vi "test11-RegisterStatusFromNonCSM_State.vi"(8 "error in (no error)":errorcluster, 11 "TestCase in":refnum<class "testcase-CSMBroadcast.lvclass">) -> (0 "error out":errorcluster, 3 "TestCase out":refnum<class "testcase-CSMBroadcast.lvclass">)   [LabVIEW 2017, in "testcase-CSMBroadcast.lvclass"]
uses:
  testcase-CSMBroadcast.lvclass
  <vilib>/addons/_JKI Toolkits/VI Tester/TestCase.llb/TestCase.lvclass
  src/user.lib/_NEVSTOP/Communicable State Machine(CSM)/Communicable State Machine.lvlib
  CSM/CSM-Testcase.lvlib
  C:/Program Files (x86)/National Instruments/LabVIEW 2017/vi.lib/addons/_JKI Toolkits/VI Tester/TestCase.llb/TestCase.lvclass
panel:
  out "LoopCount":i32
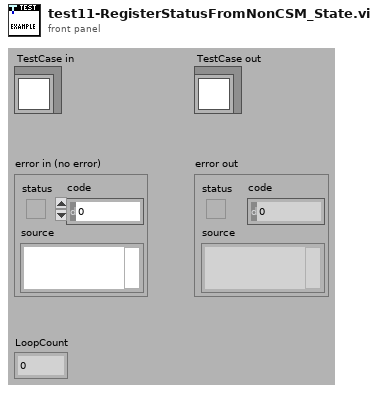
[diagram p1: front panel]
types:
  T1 = cluster{"ModuleName":string, "Status":string, "Arguments":string}
  T2 = cluster{"cluster":cluster{"ModuleName":string, "Status":string, "Arguments":string}}
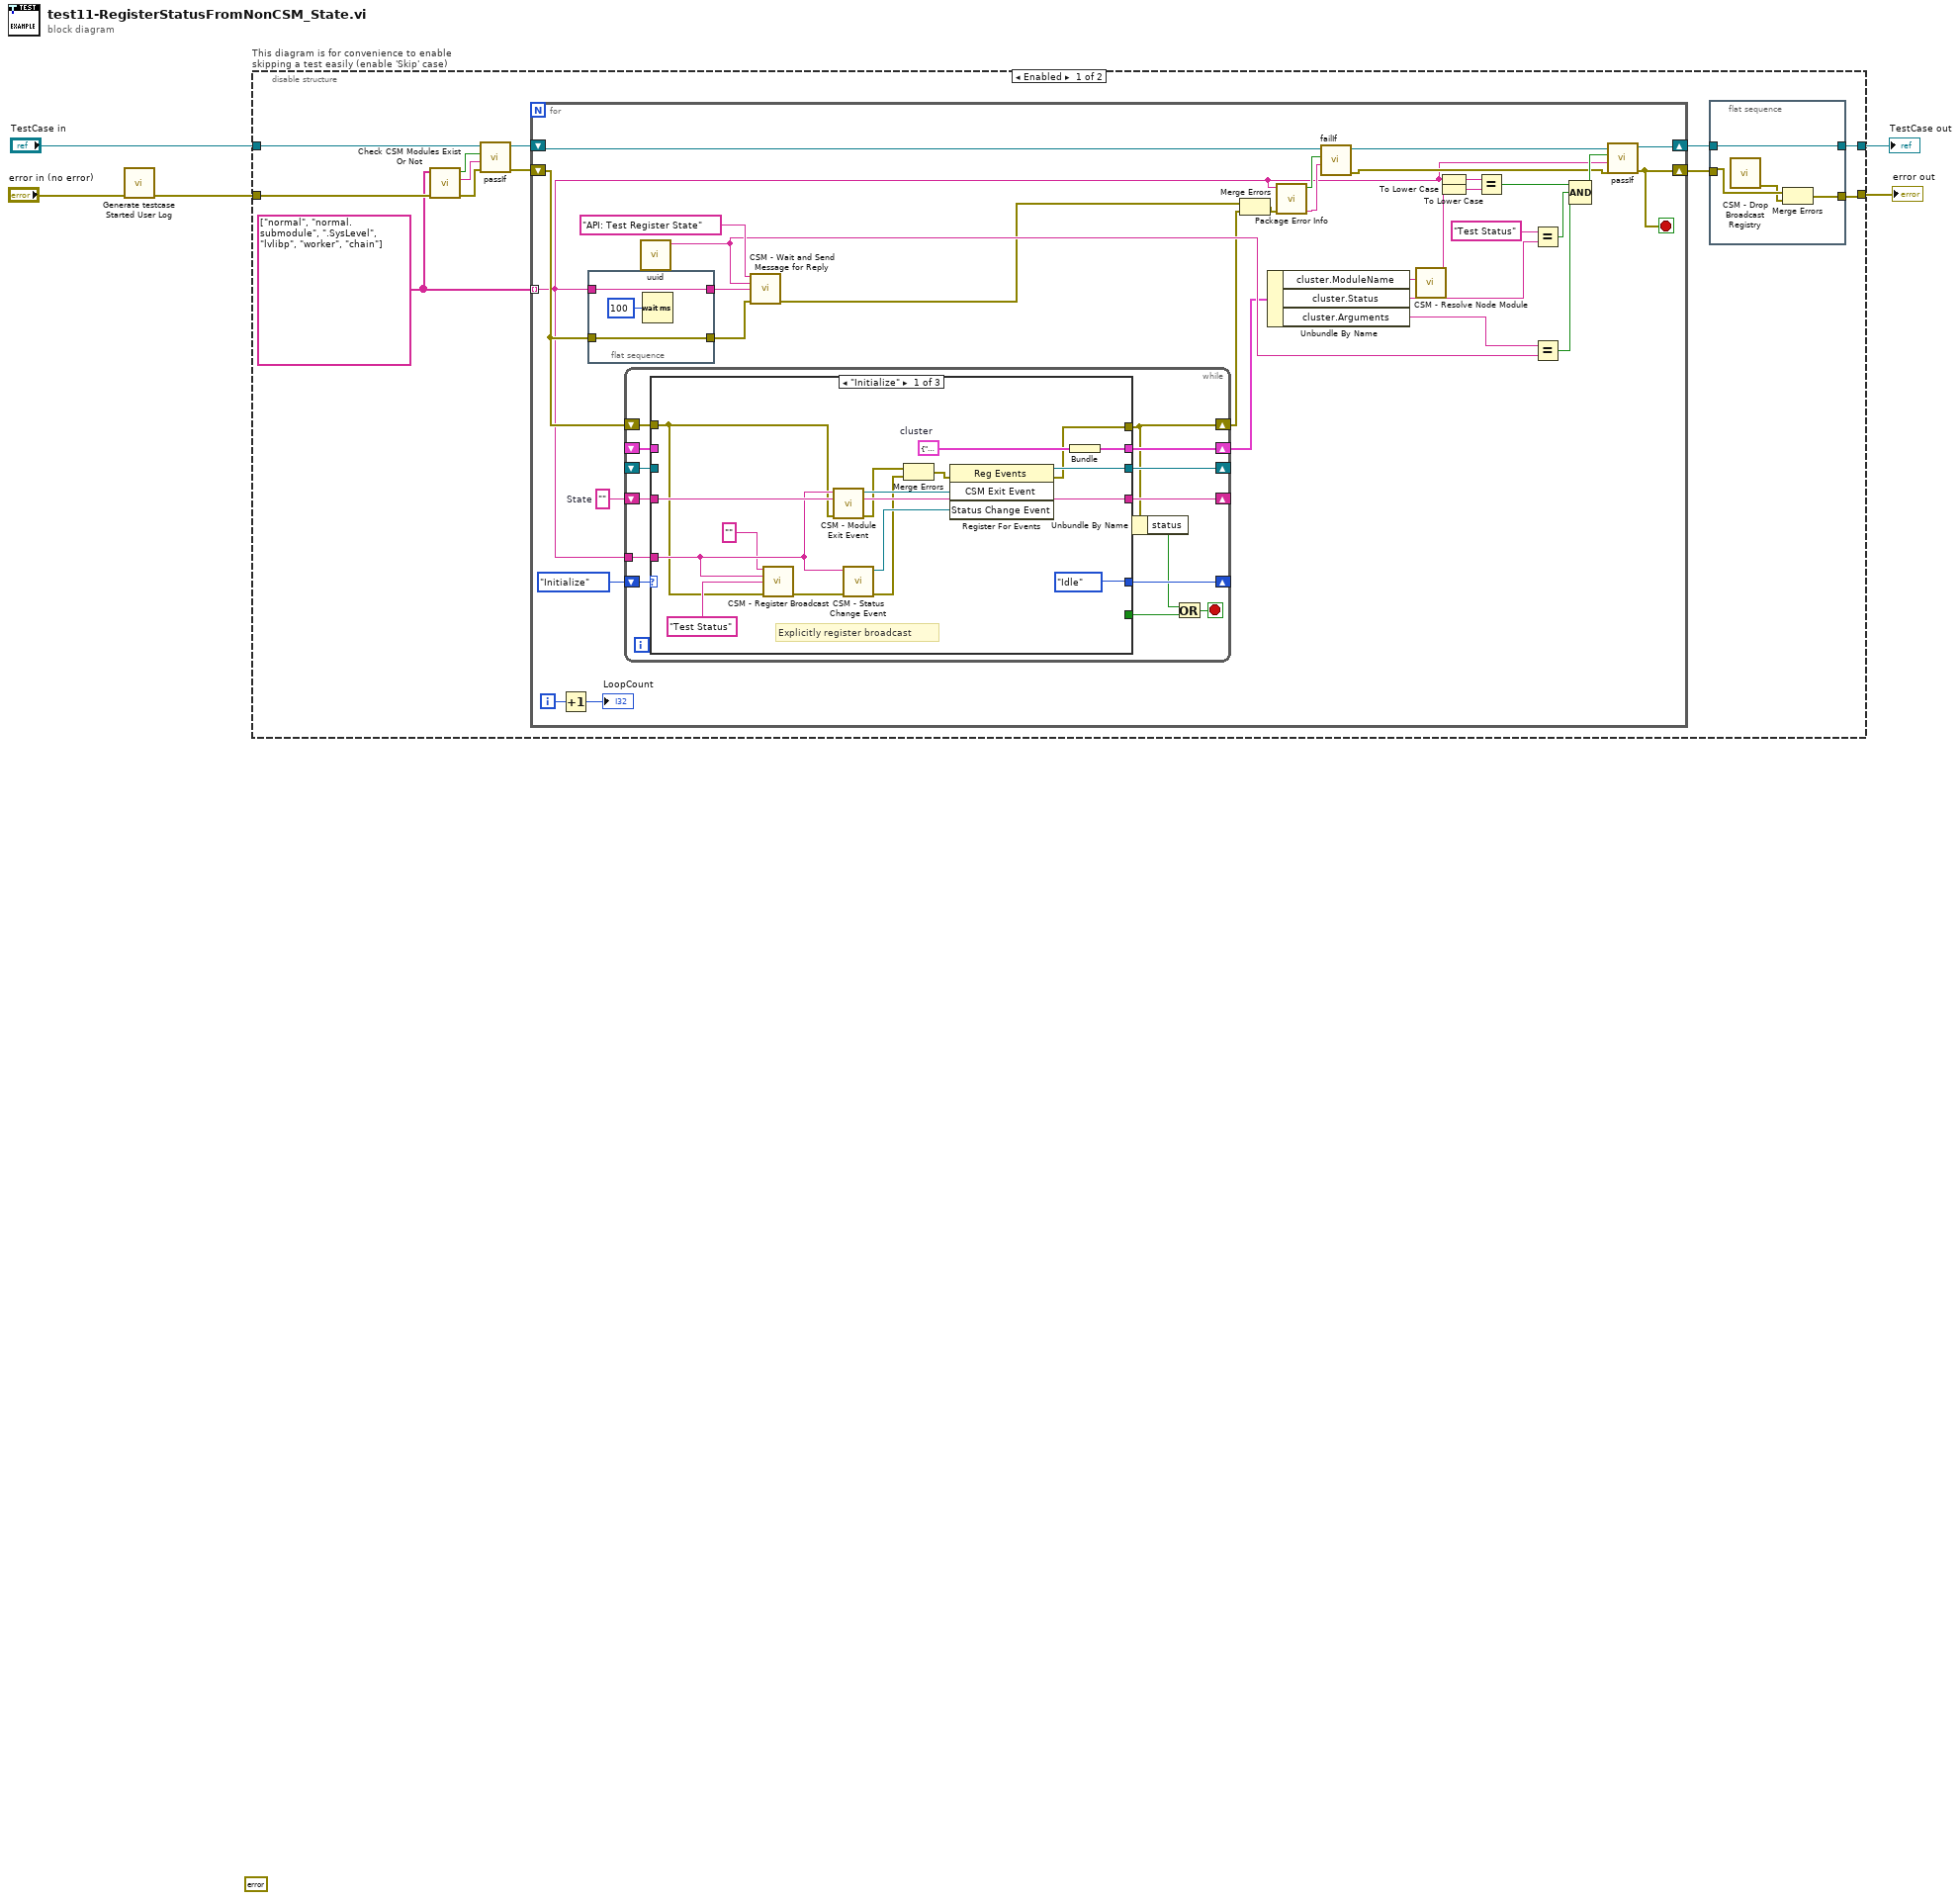
[diagram p0: block diagram]
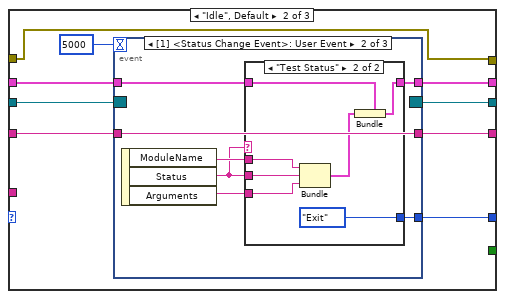
[diagram p2: hidden frame]
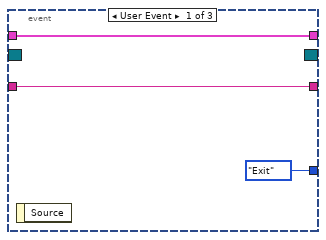
[diagram p3: hidden frame]
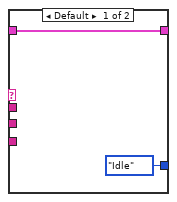
[diagram p4: hidden frame]
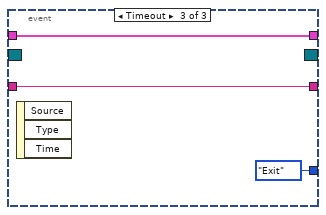
[diagram p5: hidden frame]
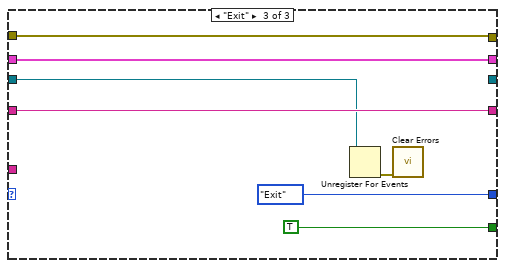
[diagram p6: hidden frame]
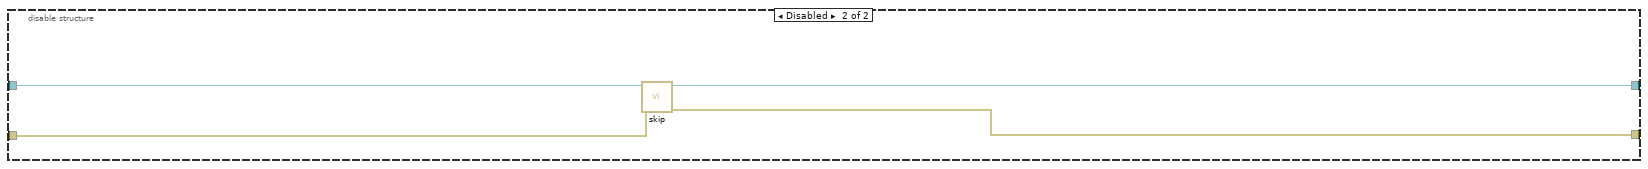
[diagram p7: hidden frame]
diagram:
  (unwired) errorcluster {"status"=FALSE, "code"=0, "source"=""} ("error out")
  n1 = call "Generate testcase Started User Log.vi"("Error In"="error in (no error)") -> ("error out"=w1:errorcluster)  [unwired: 10 in]
  n2 = disable-structure "This diagram is for convenience to enable skipping a test easily (enable 'Skip' case)" shown="Enabled" {
    disable-tunnel: "TestCase in" -> [w13 w128]
    disable-tunnel: [w7 w126] -> w3
    disable-tunnel: [w17 w127] -> w2
    disable-tunnel: w1 -> [w10 w125]
    frame Enabled {
      w9 = string[] ["normal", "normal.submodule", ".SysLevel", "lvlibp", "worker", "chain"]
      n3 = call "Check CSM Modules Exist Or Not.vi"("error in"=w10, "CSM names in"=w9) -> ("error out"=w14:errorcluster, "Debug string"=w15:string, "All Modules Exist?"=w16:bool)  [unwired: 7 in]
      n4 = call-dynamic "passIf.vi"("error in (no error)"=w14, "message (\"\")"=w15, "pass"=w16, "TestCase in"=w13) -> ("error out"=w11:errorcluster, "TestCase out"=w12:refnum<class "testcase-CSMBroadcast.lvclass">)  [unwired: 6 in]
      n5 = for {
        shift-right: [w45] -> w8
        shift-left: w12 -> [w29]
        tunnel: w9 -> [w24] mode=indexing
        shift-right: [w38] -> w6
        shift-left: w11 -> [w31]
        i -> [w40]
        stop <- w38 stop-if-true
        w52 = ""  # State
        n6 = Increment(x=w40) -> (x+1=→"LoopCount":i32)
        n7 = flat-sequence {
          tunnel: w24 -> [w56]
          tunnel: [w56] -> w50
          tunnel: w31 -> [w54]
          tunnel: [w54] -> w32
          frame #0 {
            n8 = Wait (ms)(milliseconds to wait=u32 100) -> ()  [unwired: 1 out]
          }
        }
        n9 = while {
          shift-right: [w69] -> _
          shift-left: enum16{"Idle", "Initialize", "Exit"}."Initialize" -> [w70]
          shift-right: [w67] -> _
          shift-left: w52 -> [w68]
          shift-right: [w66] -> _
          shift-left: _ -> [w65]
          shift-right: [w64] -> w37
          shift-left: _ -> [w63]
          tunnel: w24 -> [w62]
          shift-right: [w58] -> w26
          shift-left: w31 -> [w61]
          stop <- w60 stop-if-true
          n10 = case shown="\"Initialize\"" w70 {
            tunnel: [enum16{"Idle", "Initialize", "Exit"}."Idle" w95 enum16{"Idle", "Initialize", "Exit"}."Exit"] -> w69
            tunnel: [_ _ TRUE] -> w59
            tunnel: w68 -> [w85 w93 w122]
            tunnel: [w85 w94 w122] -> w67
            tunnel: [w83 w91 _] -> w66
            tunnel: w65 -> [_ w92 w121]
            tunnel: [w82 w89 w119] -> w64
            tunnel: w63 -> [_ w90 w119]
            tunnel: w62 -> [w76 _ _]
            tunnel: w61 -> [w73 w87 w118]
            tunnel: [w71 w87 w118] -> w58
            frame "Initialize" {
              w80 = T1 {"ModuleName"="", "Status"="", "Arguments"=""}  # cluster
              # "Explicitly register broadcast"
              n11 = call "CSM - Register Broadcast.vi"("CSM Name(Empty for Broadcast Event)"="", "Source CSM Name (* as Default)"=w76, "Trigger"="Test Status" ("State"), "Error In"=w73) -> ("error out"=w77:errorcluster)  [unwired: 10 in, 1 out]
              n12 = call "CSM - Module Exit Event.vi"("Error In"=w73, "Name (\"\" to Use UUID) In"=w76) -> ("error out"=w79:errorcluster, "CSM Exit Event"=w84:refnum<user-event>)  [unwired: 7 in, 1 out]
              n13 = call "CSM - Status Change Event.vi"("Error In"=w77, "CSM Module"=w76) -> ("error out"=w78:errorcluster, "Status Change Event"=w81:refnum<user-event>)  [unwired: 7 in, 1 out]
              n14 = Merge Errors(w79, w78) -> (w72:errorcluster)
              n15 = register-events(error in=w72, w84, w81) -> (reference out=w83:refnum<event-registration>, error out=w71:errorcluster)  [unwired: 1 in]
              n16 = Bundle("cluster"=w80) -> (w82:T2)  [unwired: 1 in]
            }
            frame "Idle", Default {
              n17 = event shown="[1] <Status Change Event>: User Event" {
                selector: w92 -> [_ _ _]
                dyn-events: [_ _ _] -> w91
                timeout: 5000 -> [_ _ _]
                tunnel: [enum16{"Idle", "Initialize", "Exit"}."Exit" w104 enum16{"Idle", "Initialize", "Exit"}."Exit"] -> w95
                tunnel: w93 -> [w98 w105 w117]
                tunnel: [w98 w105 w117] -> w94
                tunnel: w90 -> [w96 w101 w116]
                tunnel: [w96 w100 w116] -> w89
                event User Event {
                  n18 = event-data() -> ()  [unwired: 1 in, 1 out]
                }
                event User Event {
                  n19 = event-data() -> ("ModuleName"=w103:string, "Status"=w99:string, "Arguments"=w102:string)  [unwired: 1 in]
                  n20 = case shown="\"Test Status\"" w99 {
                    tunnel: [enum16{"Idle", "Initialize", "Exit"}."Idle" enum16{"Idle", "Initialize", "Exit"}."Exit"] -> w104
                    tunnel: w103 -> [_ w113]
                    tunnel: w99 -> [_ w112]
                    tunnel: w102 -> [_ w111]
                    tunnel: w101 -> [w107 w110]
                    tunnel: [w107 w108] -> w100
                    frame Default {
                    }
                    frame "Test Status" {
                      n21 = Bundle("ModuleName"=w113, "Status"=w112, "Arguments"=w111) -> (w109:T1)  [unwired: 1 in]
                      n22 = Bundle(cluster=w110, "cluster"=w109) -> (w108:T2)
                    }
                  }
                }
                event Timeout {
                  n23 = event-data() -> ()  [unwired: 1 in, 3 out]
                }
              }
            }
            frame "Exit" {
              n24 = Unregister For Events(event registration refnum=w121) -> (error out=w120:errorcluster)  [unwired: 1 in]
              n25 = call <vilib>:"Clear Errors.vi"("error in (no error)"=w120) -> ()  [unwired: 5 in, 2 out]
            }
          }
          n26 = Unbundle By Name(w58) -> ("status"=w57:bool)
          n27 = Or(x=w57, y=w59) -> (x .or. y?=w60:bool)
        }
        n28 = call "uuid.vi"() -> ("UUID"=w47:string)  [unwired: 11 in]
        n29 = call "CSM - Wait and Send Message for Reply.vi"("State"="API: Test Register State", "Arguments (\"\")"=w47, "Target Module"=w50, "Error In (No Error)"=w32) -> ("error out"=w22:errorcluster)  [unwired: 8 in, 3 out]
        n30 = Merge Errors(w22, w26) -> (w23:errorcluster)
        n31 = Unbundle By Name(w37) -> ("cluster.ModuleName"=w35:string, "cluster.Status"=w48:string, "cluster.Arguments"=w46:string)
        n32 = call "Package Error Info.vi"("error in"=w23, "String in"=w24) -> ("packed error info out"=w27:string, "error status"=w30:bool)  [unwired: 8 in]
        n33 = call-dynamic "failIf.vi"("message (\"\")"=w27, "fail"=w30, "TestCase in"=w29) -> ("error out"=w25:errorcluster, "TestCase out"=w28:refnum<class "testcase-CSMBroadcast.lvclass">)  [unwired: 7 in]
        n34 = call "CSM - Resolve Node Module.vi"("Node Name"=w35) -> ("CSM Module Name"=w33:string)  [unwired: 10 in]
        n35 = To Lower Case(string=w24) -> (all lower case string=w36:string)
        n36 = To Lower Case(string=w33) -> (all lower case string=w34:string)
        n37 = Equal?(x=w36, y=w34) -> (x = y?=w44:bool)
        n38 = Equal?(x="Test Status" ("State"), y=w48) -> (x = y?=w43:bool)
        n39 = Equal?(x=w46, y=w47) -> (x = y?=w42:bool)
        n40 = Compound Arithmetic op=AND(w44, w43, w42) -> (w41:bool)
        n41 = call-dynamic "passIf.vi"("error in (no error)"=w25, "message (\"\")"=w24, "pass"=w41, "TestCase in"=w28) -> ("error out"=w38:errorcluster, "TestCase out"=w45:refnum<class "testcase-CSMBroadcast.lvclass">)  [unwired: 6 in]
      }
      n42 = flat-sequence {
        tunnel: w6 -> [w21]
        tunnel: [w20] -> w17
        tunnel: w8 -> [w19]
        tunnel: [w19] -> w7
        frame #0 {
          n43 = call "CSM - Drop Broadcast Registry.vi"() -> ("error out"=w18:errorcluster)  [unwired: 15 in]
          n44 = Merge Errors(w21, w18) -> (w20:errorcluster)
        }
      }
    }
    frame Disabled {
      # "skip test result while test is under development"
      n45 = call <vilib>:"skip.vi"("error in (no error)"=w125, "TestCase in"=w128) -> ("error out"=w127:errorcluster, "TestCase out"=w126:refnum<class "testcase-CSMBroadcast.lvclass">)  [unwired: 8 in]
    }
  }
  "error out" <- w2
  "TestCase out" <- w3
